vi "Send Transfer Group.vi"(7 "Command":T1=enum."Tx", 8 "error in (no error)":errorcluster, 10 "Transfer Group in":refnum<class "Transfer Group.lvclass">, 11 "Plugin in":refnum<class "Plugin.lvclass">) -> (0 "error out":errorcluster, 2 "Transfer Group out":refnum<class "Transfer Group.lvclass">, 3 "Plugin out":refnum<class "Plugin.lvclass">)   [LabVIEW 2017, in "DSF Core.lvlib" / "Plugin.lvclass"]
uses:
  Plugin.lvclass
  Transfer Group/Transfer Group.lvclass
  Interfaces/Transceiver Interface/Command.ctl
  Interfaces/Transceiver Interface/Plugin Interface.lvclass
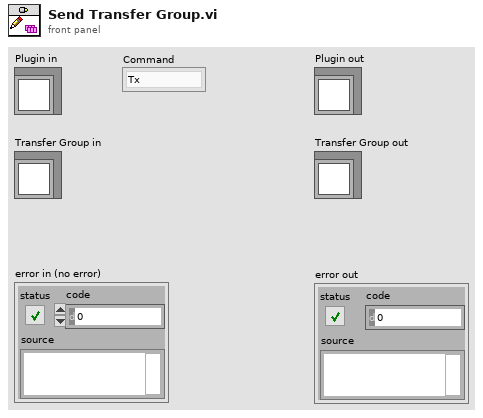
[diagram p1: front panel]
types:
  T1 = typedef "DSF Core.lvlib/Plugin Interface.lvclass/Command.ctl" = enum8{"Set Inline Buffer", "Rx", "Tx", "Shutdown"}
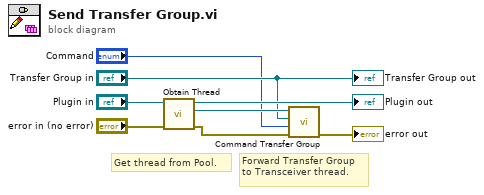
[diagram p0: block diagram]
diagram:
  # "Forward Transfer Group to Transceiver thread."
  # "Get thread from Pool."
  n1 = call "Obtain Thread.vi"("error in (no error)"="error in (no error)", "Plugin in"="Plugin in") -> ("error out"=w6:errorcluster, "Plugin Thread Interface"=w7:refnum<class "Plugin Interface.lvclass">, "Plugin out"=→"Plugin out":refnum<class "Plugin.lvclass">)  [unwired: 7 in]
  n2 = call "Command Transfer Group.vi"("error in (no error)"=w6, "Command"="Command", "Transfer Group"="Transfer Group in", "Plugin Interface in"=w7) -> ("error out"=→"error out":errorcluster)  [unwired: 6 in, 1 out]
  "Transfer Group out" <- "Transfer Group in"
